vi "Run Unit Tests.vi"(8 "Error In":errorcluster) -> (0 "Error Out":errorcluster)   [LabVIEW 2017, in "Scripts.lvlib"]
uses:
  Scripts.lvlib
  <vilib>/addons/_JKI Toolkits/Caraya/classes/Test/Test.lvclass
  Toolkit/Tests/Tests.lvlib
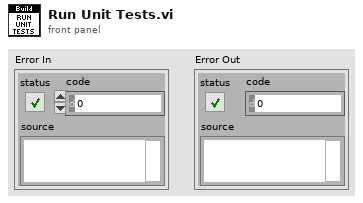
[diagram p1: front panel]
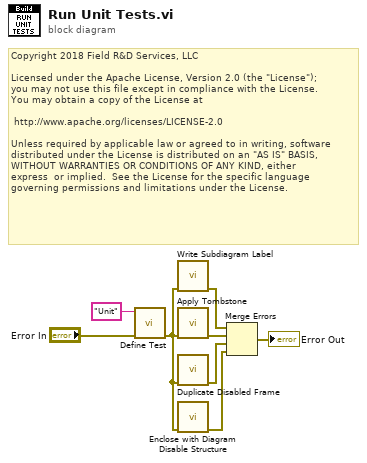
[diagram p0: block diagram]
diagram:
  # "Copyright 2018 Field R&D Services, LLC\n\nLicensed under the Apache License, Version 2.0 (the \"License\");\nyou may not use this file except in compliance with the License.\nYou may obtain a copy of the License at\n\n\thttp://www.apache.org/licenses/LICENSE-2.0\n\nUnless required by applicable law or agreed to in writing, software\ndistributed under the License is distributed on an \"AS IS\" BASIS,\nWITHOUT WARRANTIES OR CONDITIONS OF ANY KIND, either \nexpress  or implied.  See the License for the specific language \ngoverning permissions and limitations under the License."
  n1 = call <vilib>:"Define Test.vi"("error in (no error)"="Error In", "Label (VI Title)"="Unit") -> ("error out"=w2:errorcluster)  [unwired: 9 in]
  n2 = call "Write Subdiagram Label.vi"("Error In"=w2) -> ("Error Out"=w6:errorcluster)  [unwired: 10 in]
  n3 = call "Apply Tombstone.vi"("Error In"=w2) -> ("Error Out"=w4:errorcluster)  [unwired: 10 in]
  n4 = call "Duplicate Disabled Frame.vi"("Error In"=w2) -> ("Error Out"=w3:errorcluster)  [unwired: 10 in]
  n5 = call "Enclose with Diagram Disable Structure.vi"("Error In"=w2) -> ("Error Out"=w1:errorcluster)  [unwired: 10 in]
  n6 = Merge Errors(w6, w4, w3, w1) -> (→"Error Out":errorcluster)
